vi "배열최소최대...합...160329.vi"() -> ()   [LabVIEW 2014]
panel:
  out "최소값":dbl
  out "최대값":dbl
  out "합계":dbl
  out "숫자형 2":dbl
  out "숫자형":dbl
  out "배열":dbl[](array[numeric])
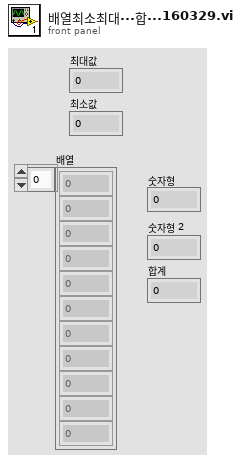
[diagram p1: front panel]
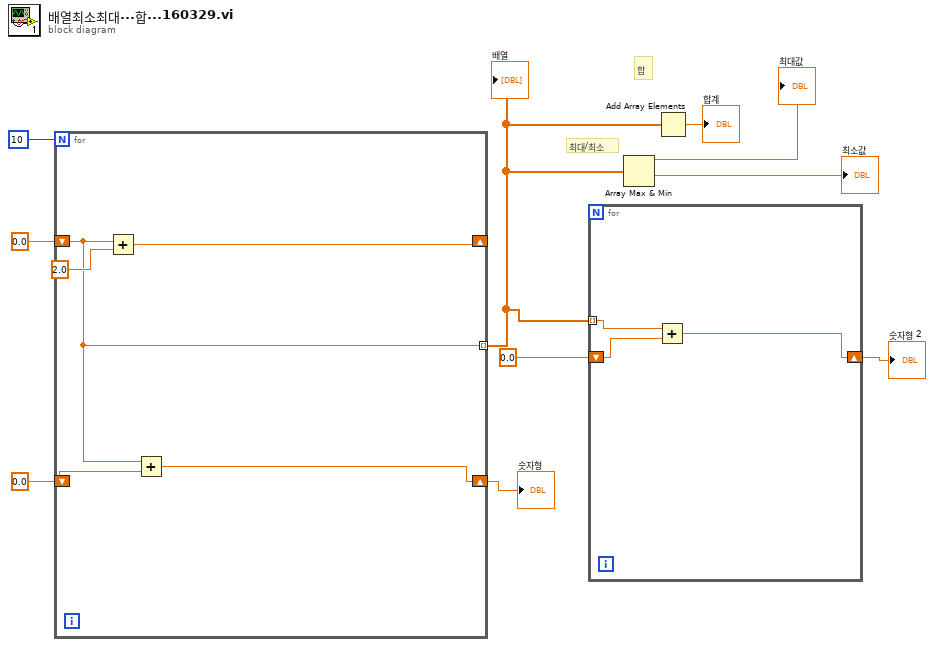
[diagram p0: block diagram]
diagram:
  # "최대/최소"
  # "합"
  n1 = for {
    N: 10 -> [_]
    shift-right: [w15] -> _
    shift-left: 0.0 -> [w13]
    tunnel: [w13] -> w3 mode=indexing
    shift-right: [w11] -> w8
    shift-left: 0.0 -> [w12]
    n2 = Add(x=w13, y=2.0) -> (x+y=w15:dbl)
    n3 = Add(x=w13, y=w12) -> (x+y=w11:dbl)
  }
  "배열" <- w3
  "숫자형" <- w8
  n4 = for {
    tunnel: w3 -> [w18] mode=indexing
    shift-right: [w16] -> w5
    shift-left: 0.0 -> [w17]
    n5 = Add(x=w18, y=w17) -> (x+y=w16:dbl)
  }
  "숫자형 2" <- w5
  n6 = Array Max & Min(array=w3) -> (max value=→"최대값":dbl, min value=→"최소값":dbl)  [unwired: 2 out]
  n7 = Add Array Elements(numeric array=w3) -> (sum=→"합계":dbl)
